vi "Generate pulse train.vi"(4 "Pulse division settings in":u32[](array[numeric])=[0, 0, 0, 0] min=1 step=1, 5 "Pulse train length (ticks) in":u32, 6 "Channel accumulators in":u32[](array[numeric])=[0, 0, 0, 0], 7 "Channel timings (ticks) in":u32[](array[numeric])=[0, 0, 0, 0], 8 "Pulses enabled?":bool, 10 "Channels on/off":bool[](array[boolean])=[FALSE, FALSE, FALSE, FALSE], 11 "Pulse width (ticks)":u32) -> (1 "Channel accumulators out":u32[](array[numeric]))   [LabVIEW 2013]
doc: "This SubVI generates the pulse train using the NI 9401 module. The pulse train is accurate to a single FPGA clock cycle.\n\nThe generator runs in a single-cycle timed loop. With a 40MHz clock, this gives us a timing resolution of 25ns per tick. The quoted jitter for a CompactRIO is a few hundred picoseconds.\n\nWhile the tick number is less than (pulse train length-1), generate the pulses for 4 channels. The implementation details for the pulse generation are documented in detail in \"FPGA channel logic.vi\".\n\nWhen the tick number equals (pulse train length-1), we've reached the end of the pulse train. All outputs should have been set LOW, but just to be on the safe side set all outputs LOW explicitly."
uses:
  <vilib>/Platform/TimedLoop/XDataNode/timing_clust.ctl
  <vilib>/Platform/TimedLoop/XDataNode/nitl_modes.ctl
  <vilib>/Platform/TimedLoop/XDataNode/wakeup.ctl
  <vilib>/rvi/Emulation/niFpgaSctlEmulationGetInTimedLoop.vi
  <vilib>/rvi/Emulation/niFpgaEmulationReportErrorSimple.vi
  <vilib>/rvi/Emulation/niFpgaGetClockAttributes.vi
  <vilib>/rvi/Emulation/niFpgaCriticalErrorInLSC.vi
  <vilib>/rvi/eio/common/nirviEmuTemplateMethod_errors.vi
  <vilib>/Platform/TimedLoop/XDataNode/XDataNode.xnode
  <vilib>/eio/EIONode/EIONode.xnode
  <vilib>/Platform/TimedLoop/XDataNode/XDNodeRunTimeDep.lvlib
panel:
  # "Generate pulse train"
  # "Generates timed hardware signals accurate to a single FPGA clock cycle."
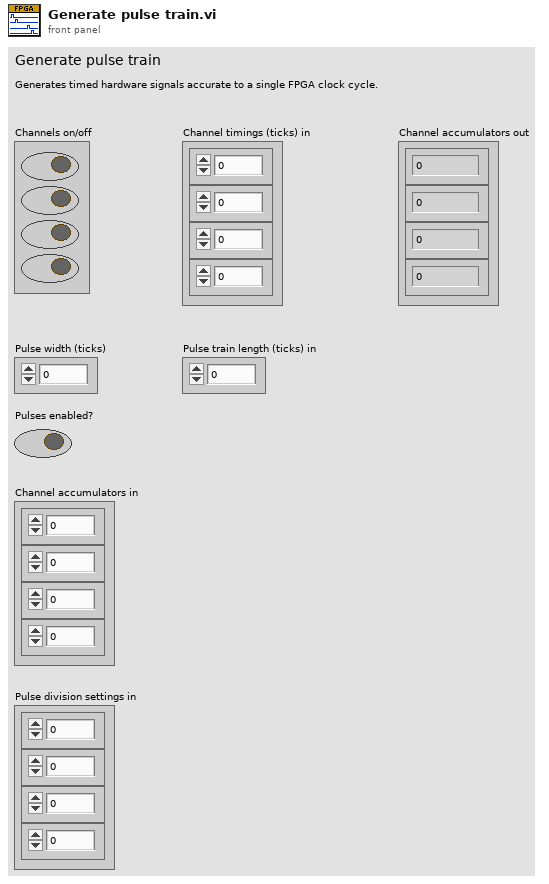
[diagram p1: front panel]
types:
  T1 = typedef "XDNodeRunTimeDep.lvlib/timing_clust.ctl" = cluster{"Expected End [f-1]":u64, "Actual End [f-1]":u64, "Finished Late? [f-1]":bool, "Expected End [i-1]":u64, "Actual End [i-1]":u64, "Finished Late? [i-1]":bool, "Expected Start [i]":u64, "Actual Start [i]":u64, "Expected Start [f]":u64, "Actual Start [f]":u64, "Source Name":string, "Structure Name":string, "Period":i64, "Deadline":i64, "Offset":i64, "Start":i64, "Priority":i32, "Timeout":i32, "Mode":T2, "Wakeup Reason":T3, "Error":errorcluster, "Source Type":string, "Secondary Source Type":string, "Global End Time":u64, "Global Start Time":u64, "Frame Duration":u64, "Iteration Duration":u64, "Assigned CPU":i32, "I/O Scan Engine Mode":u32}
  T2 = typedef "XDNodeRunTimeDep.lvlib/nitl_modes.ctl" = enum32{"No Change", "Process missed periods, maintain original phase", "Discard missed periods, maintain original phase", "Process missed periods, ignore original phase", "Discard missed periods, ignore original phase"}
  T3 = typedef "XDNodeRunTimeDep.lvlib/wakeup.ctl" = enum32{"Normal", "Aborted", "Asynchronous wakeup", "Timing source error", "Timed loop error", "Timeout"}
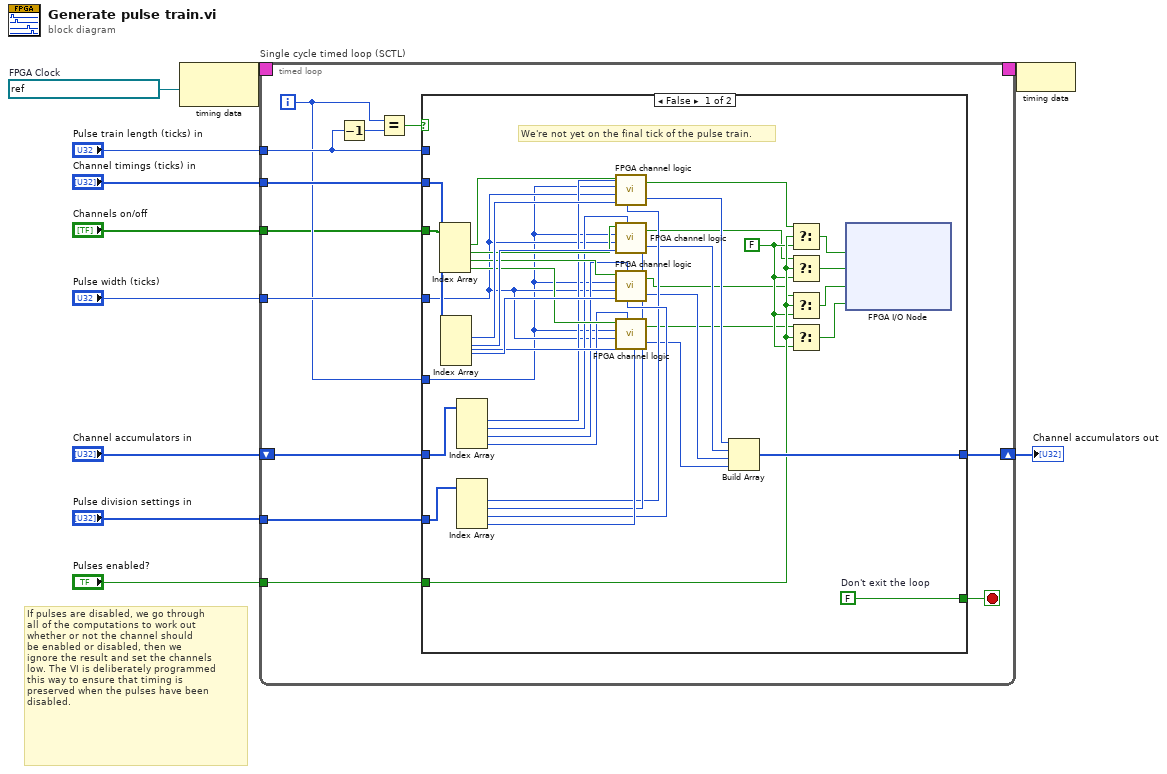
[diagram p0: block diagram]
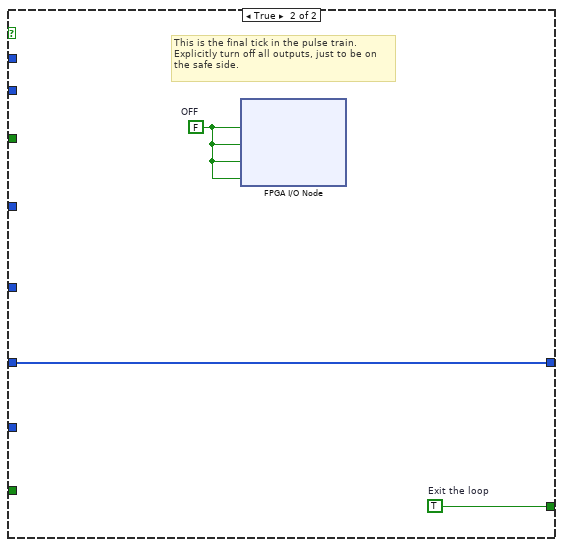
[diagram p2: hidden frame]
diagram:
  w1 = refnum<k21> "40 MHz Onboard Clock"  # FPGA Clock
  # "If pulses are disabled, we go through \nall of the computations to work out \nwhether or not the channel should\nbe enabled or disabled, then we \nignore the result and set the channels\nlow. The VI is deliberately programmed\nthis way to ensure that timing is\npreserved when the pulses have been\ndisabled."
  n1 = node-c288(w1) -> (w11:T1)
  n2 = timed-loop "Single cycle timed loop (SCTL)" {
    tunnel: "Pulse width (ticks)" -> [w21]
    timing: w11 -> [_]
    timing-out: [_] -> w10
    tunnel: "Channels on/off" -> [w16]
    tunnel: "Pulse division settings in" -> [w14]
    shift-right: [w13] -> w8
    shift-left: "Channel accumulators in" -> [w15]
    tunnel: "Pulse train length (ticks) in" -> [w22]
    tunnel: "Pulses enabled?" -> [w12]
    tunnel: "Channel timings (ticks) in" -> [w23]
    i -> [w17]
    stop <- w18 stop-if-true
    n3 = Decrement(x=w22) -> (x-1=w19:u32)
    n4 = Equal?(x=w17, y=w19) -> (x = y?=w20:bool)
    n5 = case shown="False" w20 {
      tunnel: w17 -> [w34 _]
      tunnel: w22 -> [_ _]
      tunnel: w23 -> [w61 _]
      tunnel: w21 -> [w35 _]
      tunnel: [w56 w64] -> w18
      tunnel: w16 -> [w55 _]
      tunnel: w15 -> [w50 w63]
      tunnel: w14 -> [w36 _]
      tunnel: [w37 w63] -> w13
      tunnel: w12 -> [w33 _]
      frame False {
        w30 = FALSE ("f")
        w56 = FALSE  # Don't exit the loop
        # "We're not yet on the final tick of the pulse train."
        n6 = Index Array(array=w55) -> (element #1=w54:bool, element #2=w53:bool, element #3=w52:bool, element #4=w51:bool)  [unwired: 4 in]
        n7 = Index Array(array=w61) -> (element #1=w60:u32, element #2=w59:u32, element #3=w58:u32, element #4=w57:u32)  [unwired: 4 in]
        n8 = Index Array(array=w50) -> (element #1=w49:u32, element #2=w48:u32, element #3=w47:u32, element #4=w46:u32)  [unwired: 4 in]
        n9 = Index Array(array=w36) -> (element #1=w42:u32, element #2=w43:u32, element #3=w44:u32, element #4=w45:u32)  [unwired: 4 in]
        n10 = call "FPGA channel logic.vi"("Pulse divide"=w42, "Accumulator in"=w49, "Channel ON at tick"=w60, "Pulse width (ticks)"=w35, "Current tick number"=w34, "Channel enabled?"=w54) -> ("Accumulator out"=w41:u32, "Channel ON/OFF"=w32:bool)
        n11 = call "FPGA channel logic.vi"("Pulse divide"=w43, "Accumulator in"=w48, "Channel ON at tick"=w59, "Pulse width (ticks)"=w35, "Current tick number"=w34, "Channel enabled?"=w53) -> ("Accumulator out"=w40:u32, "Channel ON/OFF"=w29:bool)
        n12 = call "FPGA channel logic.vi"("Pulse divide"=w44, "Accumulator in"=w47, "Channel ON at tick"=w58, "Pulse width (ticks)"=w35, "Current tick number"=w34, "Channel enabled?"=w52) -> ("Accumulator out"=w39:u32, "Channel ON/OFF"=w27:bool)
        n13 = call "FPGA channel logic.vi"("Pulse divide"=w45, "Accumulator in"=w46, "Channel ON at tick"=w57, "Pulse width (ticks)"=w35, "Current tick number"=w34, "Channel enabled?"=w51) -> ("Accumulator out"=w38:u32, "Channel ON/OFF"=w25:bool)
        n14 = Build Array(w41, w40, w39, w38) -> (w37:u32[])
        n15 = Select(t=w32, s=w33, f=w30) -> (s? t:f=w31:bool)
        n16 = Select(t=w29, s=w33, f=w30) -> (s? t:f=w28:bool)
        n17 = Select(t=w27, s=w33, f=w30) -> (s? t:f=w26:bool)
        n18 = Select(t=w25, s=w33, f=w30) -> (s? t:f=w24:bool)
        n19 = xnode "FPGA I/O Node"("Mod1/DIO0"=w31, "Mod1/DIO1"=w28, "Mod1/DIO2"=w26, "Mod1/DIO3"=w24) -> ()  [unwired: 4 in, 4 out]
      }
      frame True {
        w64 = TRUE  # Exit the loop
        w62 = FALSE  # OFF
        # "This is the final tick in the pulse train.\nExplicitly turn off all outputs, just to be on\nthe safe side."
        n20 = xnode "FPGA I/O Node"("Mod1/DIO0"=w62, "Mod1/DIO1"=w62, "Mod1/DIO2"=w62, "Mod1/DIO3"=w62) -> ()  [unwired: 4 in, 4 out]
      }
    }
  }
  "Channel accumulators out" <- w8
  n21 = node-c288(w10) -> ()
